vi "Trace.vi"(0 "Execution Unit Implementation in":refnum<class "Execution Unit.lvclass">, 1 "message":string, 3 "error in (no error)":errorcluster) -> (7 "Execution Unit Implementation out":refnum<class "Execution Unit.lvclass">, 10 "error out":errorcluster)   [LabVIEW 2020, in "Ballard MIL-STD-1553 Engine.lvlib" / "Implementation.lvlib" / "Execution Unit.lvclass"]
uses:
  Execution Unit.lvclass
  Execution Unit.lvclass/Execution Unit.ctl
  <vilib>/Utility/SystemLogging/NI_SystemLogging.lvlib
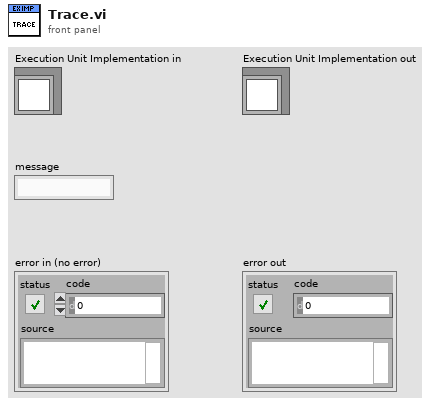
[diagram p1: front panel]
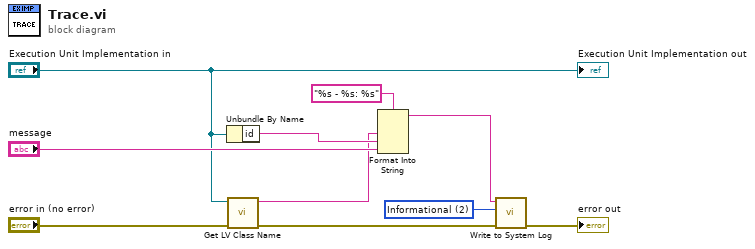
[diagram p0: block diagram]
diagram:
  w8 = 2 items=["Error", "Warning", "Informational"] ("severity")
  n1 = Unbundle By Name("Execution Unit Implementation in") -> ("id"=w2:string)
  n2 = call <vilib>:"Get LV Class Name.vi"("error in (no error)"="error in (no error)", "object"="Execution Unit Implementation in") -> ("error out"=w4:errorcluster, "class name"=w1:string)  [unwired: 8 in]
  n3 = Format Into String(format string="%s - %s: %s", w1, w2, "message") -> (resulting string=w9:string)  [unwired: 2 in, 1 out]
  n4 = call <vilib>:"Write to System Log.vi"("error in (no error)"=w4, "severity"=w8, "message"=w9) -> ("error out"=→"error out":errorcluster)  [unwired: 8 in]
  "Execution Unit Implementation out" <- "Execution Unit Implementation in"
